vi "Software Update HCC Compile Active Station List.vi"(8 "Error In":errorcluster, 11 "Station And Board ID Path":path) -> (0 "Error Out":errorcluster, 1 "List of Stations":string[][](array[string]), 2 "All Station Labels":string[](array[string]))   [LabVIEW 2016]
uses:
  <vilib>/Utility/file.llb/Read Delimited Spreadsheet (string).vi
panel:
  out "all rows":string[][](array[string])
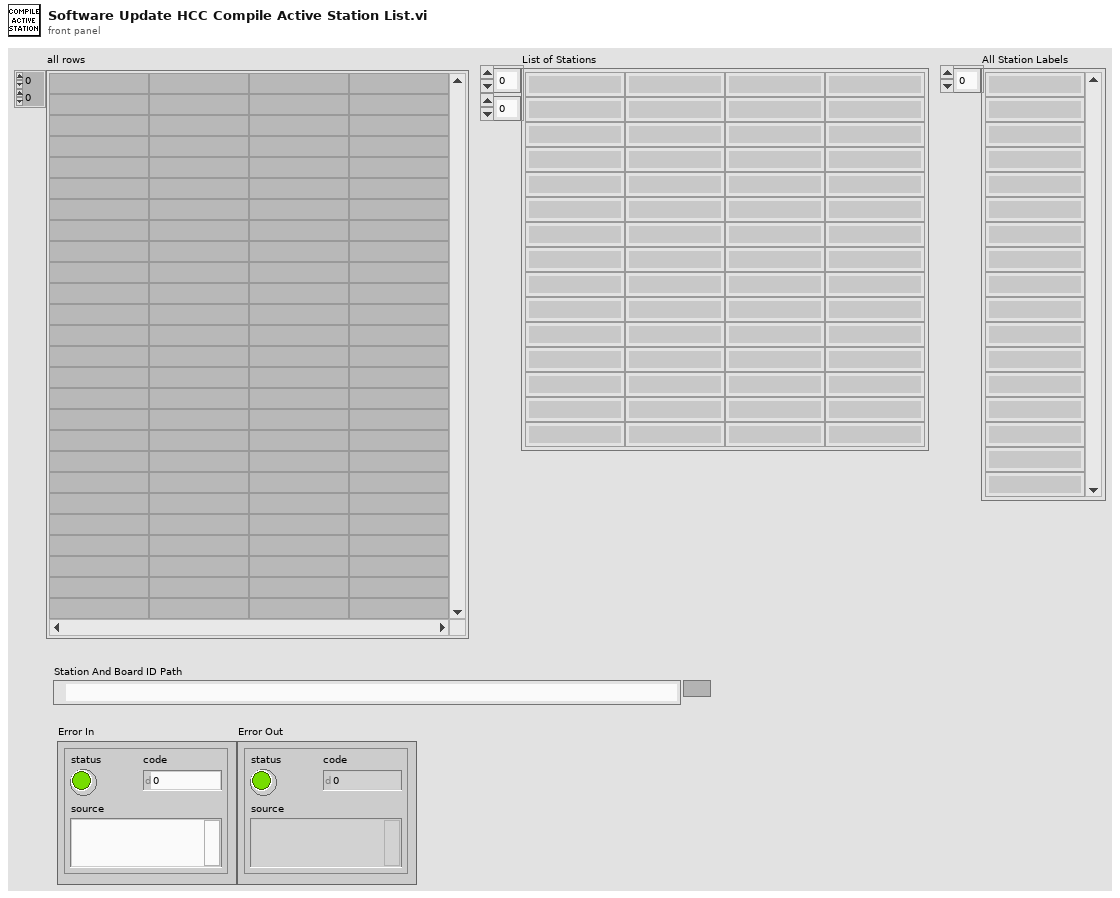
[diagram p1: front panel]
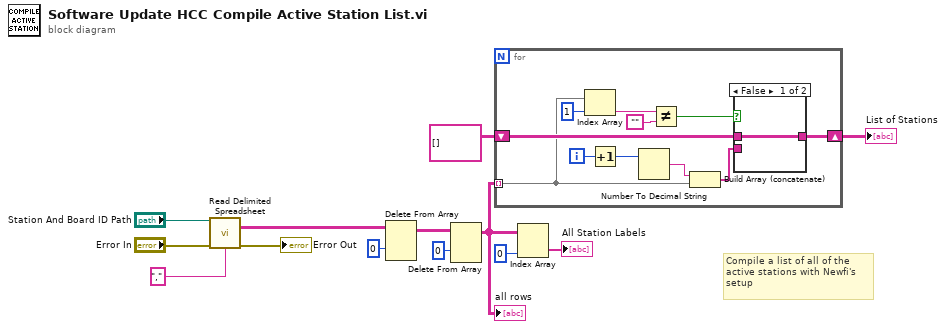
[diagram p0: block diagram]
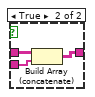
[diagram p2: hidden frame]
diagram:
  # "Compile a list of all of the \nactive stations with Newfi's \nsetup"
  n1 = call-poly <vilib>:"Read Delimited Spreadsheet.vi"("file path (dialog if empty)"="Station And Board ID Path", "error in (no error)"="Error In", "delimiter (\\t)"="," ("delimiter (\\t)")) -> ("all rows"=w5:string[][], "error out"=→"Error Out":errorcluster)  [unwired: 7 in, 4 out]
  n2 = Delete From Array(array=w5, index (row)=0) -> (array with subset deleted=w6:string[][])  [unwired: 2 in, 1 out]
  n3 = Delete From Array(array=w6, index (row)=0) -> (array with subset deleted=w11:string[][])  [unwired: 2 in, 1 out]
  "all rows" <- w11
  n4 = for {
    tunnel: w11 -> [w16] mode=indexing
    shift-right: [w19] -> w10
    shift-left: string[][] [] -> [w20]
    i -> [w18]
    n5 = Index Array(array=w16, index=1) -> (element=w23:string)
    n6 = Increment(x=w18) -> (x+1=w17:i32)
    n7 = Number To Decimal String(number=w17) -> (decimal integer string=w15:string)  [unwired: 1 in]
    n8 = Not Equal?(x=w23, y="") -> (x != y?=w21:bool)
    n9 = Build Array (concatenate)(w15, w16) -> (w14:string[])
    n10 = case shown="False" w21 {
      tunnel: w20 -> [w25 w28]
      tunnel: [w25 w27] -> w19
      tunnel: w14 -> [_ w26]
      frame False {
      }
      frame True {
        n11 = Build Array (concatenate)(w28, w26) -> (w27:string[][])
      }
    }
  }
  "List of Stations" <- w10
  n12 = Index Array(array=w11, index (col)=0 ("disabled index (col)")) -> (element=→"All Station Labels":string[])  [unwired: 1 in]
